vi "Process.vi"(7 "Override? (F)":bool, 9 "Values in":dbl[](array[numeric]), 10 "Disabled in":T1(array[ring]), 11 "Interlocks":T2[](array[typedef])) -> (2 "Disabled out":T1(array[ring]))   [LabVIEW 2022 SP3, in "Interlocks.lvlib"]
uses:
  Interlocks.lvlib
  Controls/Interlock.ctl
  Controls/Token Type.ctl
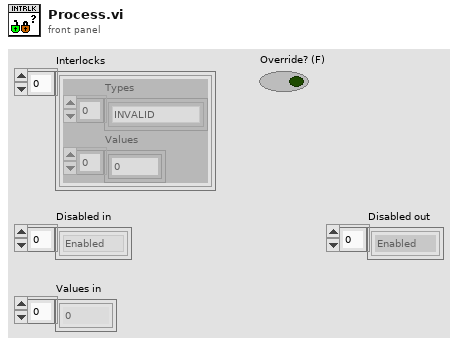
[diagram p1: front panel]
types:
  T1 = enum8{"Enabled", "Disabled", "Disabled and Grayed Out"}[]
  T2 = typedef "Interlocks.lvlib/Interlock.ctl" = cluster{"Types":T3[], "Values":dbl[]}
  T3 = typedef "Interlocks.lvlib/Token Type.ctl" = enum8{"INVALID", "NOT", "AND", "OR", "EE", "NE", "LT", "GT", "LTE", "GTE", "PLUS", "MINUS", "MULTIPLY", "DIVIDE", "MODULUS", "LPAREN", "RPAREN", "LITERAL", "IDENTIFIER", "DEFINITION"}
  T4 = enum8{"Enabled", "Disabled", "Disabled and Grayed Out"}
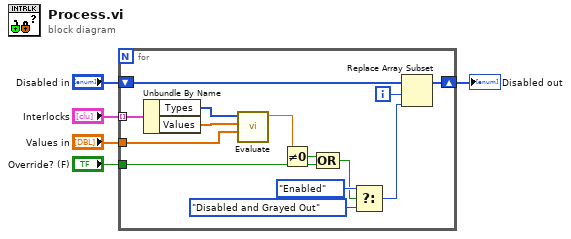
[diagram p0: block diagram]
diagram:
  n1 = for {
    tunnel: "Interlocks" -> [w19] mode=indexing
    shift-right: [w14] -> w2
    shift-left: "Disabled in" -> [w13]
    tunnel: "Override? (F)" -> [w9]
    tunnel: "Values in" -> [w6]
    i -> [w15]
    n2 = Unbundle By Name(w19) -> ("Types"=w7:T3[], "Values"=w18:dbl[])
    n3 = call "Evaluate.vi"("Variable Values"=w6, "Values"=w18, "Types"=w7) -> ("Evalulated"=w11:dbl)  [unwired: 8 in]
    n4 = Not Equal To 0?(x=w11) -> (x != 0?=w8:bool)
    n5 = Compound Arithmetic op=OR(w8, w9) -> (w10:bool)
    n6 = Select(t=T4."Enabled" ("Disabled"), s=w10, f=T4."Disabled and Grayed Out" ("Disabled")) -> (s? t:f=w12:T4)
    n7 = Replace Array Subset(array=w13, new element=w12, index=w15) -> (w14:T1)
  }
  "Disabled out" <- w2
